vi "getexpID.vi"(11 "db_File":path=path "C:/Users/YuanYuan/Desktop/Labview Data/Database") -> (0 "error out":errorcluster, 3 "data":i32)   [LabVIEW 2014, in "ChirpV2.lvclass"]
doc: "This example demonstrates how to read data from a Microsoft Access 2007 database file. You must use the ACE engine instead of the JET engine to access the database. The example database file, Access2007.accdb, is located in the labview\\examples\\database directory.\n\nRun this VI to display all the data from the example ACCDB database. Examine the block diagram of this VI to see how to use the Database Variant To Data function to convert a database variant to the data type you need."
uses:
  EIS/Electrochemical Instrument Folder/Chirp_OOP/ChirpV2.lvclass
  <vilib>/addons/database/Connection.llb/DB Tools Open Connec (String).vi
  <vilib>/addons/database/NI_Database_API.lvlib
panel:
  # "Overview: Demonstrates how to read data from a Microsoft Access 2007 database file.\nRequirements: Database Connectivity Toolkit, Office System Driver: Data Connectivity Components version 2007 or later\nInstructions:\nRun the VI to display all the data from the example ACCDB database. If an error occurs, you may need to install the Office System Driver: Data Connectivity Components version 2007 or later."
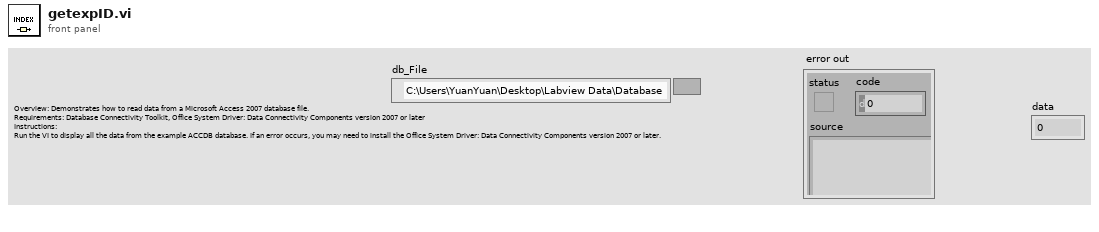
[diagram p1: front panel]
types:
  T1 = typedef "NI_Database_API.lvlib/Conn ObjectReference.ctl" = refnum<k1>
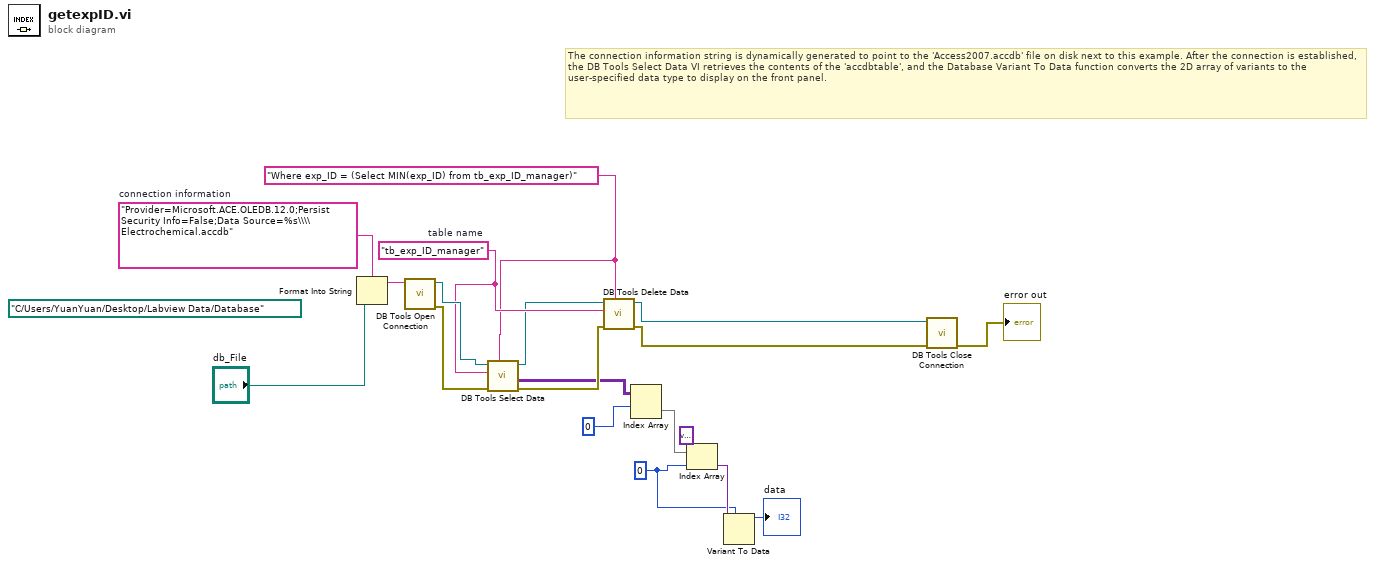
[diagram p0: block diagram]
diagram:
  (unwired) variant ("element")
  w5 = 0 ("index")
  (unwired) path "C:/Users/YuanYuan/Desktop/Labview Data/Database" ("path")
  w8 = "Where exp_ID = (Select MIN(exp_ID) from tb_exp_ID_manager)" ("condition")
  w17 = "Provider=Microsoft.ACE.OLEDB.12.0;Persist Security Info=False;Data Source=%s\\\\Electrochemical.accdb"  # connection information
  w12 = "tb_exp_ID_manager"  # table name
  # "The connection information string is dynamically generated to point to the 'Access2007.accdb' file on disk next to this example. After the connection is established, the DB Tools Select Data VI retrieves the contents of the 'accdbtable', and the Database Variant To Data function converts the 2D array of variants to the user-specified data type to display on the front panel."
  n1 = Format Into String(format string=w17, "db_File") -> (resulting string=w18:string)  [unwired: 2 in, 1 out]
  n2 = call-poly <vilib>:"DB Tools Open Connection.vi"("connection information"=w18) -> ("error out"=w11:errorcluster, "connection reference"=w13:T1)  [unwired: 7 in]
  n3 = call <vilib>:"DB Tools Select Data.vi"("condition"=w8, "error in (no error)"=w11, "table"=w12, "connection reference"=w13) -> ("error out"=w9:errorcluster, "data"=w2:variant[][], "connection reference out"=w10:T1)  [unwired: 2 in]
  n4 = call <vilib>:"DB Tools Delete Data.vi"("condition"=w8, "error in (no error)"=w9, "table"=w12, "connection reference"=w10) -> ("error out"=w14:errorcluster, "connection reference out"=w15:T1)  [unwired: 6 in]
  n5 = Index Array(array=w2, index (row)=0) -> (element=w7:variant[])  [unwired: 1 in]
  n6 = Index Array(array=w7, index=w5) -> (element=w6:variant)
  n7 = Variant To Data(type=w5, Variant=w6) -> (data=→"data":i32)  [unwired: 1 in, 1 out]
  n8 = call <vilib>:"DB Tools Close Connection.vi"("error in (no error)"=w14, "connection reference"=w15) -> ("error out"=→"error out":errorcluster)  [unwired: 5 in]
